vi "Measure EQE.vi"(6 "Skip cell?":bool, 8 "Scan settings":T1={"J-V scan"=TRUE, "J-t scan"=FALSE, "Min voltage (V)"=0.0, "Max voltage (V)"=1.4, "Step (V)"=0.01, "Measurement delay (ms)"=10.0, "1st scan FB-SC"=TRUE, "Inverted structure"=FALSE, "Stabilisation time (s)"=0.0, "Stabilisation mode"=0, "Stabilisation value (V or A) "=0.0, "Step time (s)"=1.0, "Integration time"=0, "Repeat light scans"=FALSE, "Stabilisation in the dark?"=FALSE, "J-t Min (V)"=0.0, "J-t Max (V)"=1.4, "J-t Step (V)"=0.01, "Max. power stabilisation"=FALSE, "J-t 1st scan FB-SC"=TRUE, "J-t Inverted structure"=FALSE, "Max power tracking"=FALSE, "Vmp (V)"=0.7, "Total stabilisation time (s)"=100.0, "J-t best pixel only"=0, "Max power best pixel only"=0, "Vmp from J-V scan"=FALSE, "Intensity dependence"=FALSE, "P dep best pixel only"=0, "External quantum efficiency"=FALSE, "EQE best pixel only"=0, "WL min (nm)"=300.0, "WL max (nm)"=900.0, "WL step (nm)"=5.0, "Wait (ms)"=100.0, "No. of repeat scans"=2.0, "Only repeat for best pixel"=0, "Chopper Freq.  (Hz)"=90.0, "Time Constant (s)"=2.0, "Stabilisation time step (s)"=1.0, "Illumination conditions"=2, "Scan rate min (V/s)"=0.1, "Scan rate max (V/s)"=1.0, "No. of scan rate steps"=1.0, "Scan rate voltage step priority"=FALSE, "Scan rate measurement delay priority"=FALSE, "J-t Illumination conditions"=0, "White bias  (no. of suns)"=200.0, "Max P stab. Specific voltage"=FALSE} {"J-t Illumination conditions" items=["Light only", "Dark only", "Light then dark", "Dark then light"]; "No. of scan rate steps" min=1.0 step=1.0; "Illumination conditions" items=["Light only", "Dark only", "Light then dark", "Dark then light", "Light then dark then light", "Dark then light then dark"]; "Time Constant (s)" items=["0.003", "0.01", "0.03", "0.1", "0.3", "1", "3", "10", "30", "100"]; "Only repeat for best pixel" items=["only for best pixel", "for best 2 pixels", "for best 3 pixels", "for best 4 pixels", "for best 5 pixels", "for best 6 pixels", "for best 7 pixels", "for all pixels"]; "No. of repeat scans" min=1.0 step=1.0; "EQE best pixel only" items=["only the best pixel", "the best 2 pixel", "the best 3 pixel", "the best 4 pixel", "the best 5 pixel", "the best 6 pixel", "the best 7 pixel", "all pixels"]; "P dep best pixel only" items=["only the best pixel", "the best 2 pixels", "the best 3 pixels", "the best 4 pixels", "the best 5 pixels", "the best 6 pixels", "the best 7 pixels", "all pixels"]; "Max power best pixel only" items=["only the best pixel", "the best 2 pixels", "the best 3 pixels", "the best 4 pixels", "the best 5 pixels", "the best 6 pixels", "the best 7 pixels", "all pixels"]; "J-t best pixel only" items=["only the best pixel", "the best 2 pixels", "the best 3 pixels", "the best 4 pixels", "the best 5 pixels", "the best 6 pixels", "the best 7 pixels", "all pixels"]; "Integration time" items=["Fast", "Normal", "High Accuracy"]; "Stabilisation mode" items=["V", "I"]; "Measurement delay (ms)" min=10.0}, 9 "Save data file path":string) -> (0 "Max WL (nm)":string, 1 "Min WL (nm)":string, 3 "EQE data file path":path)   [LabVIEW 2011]
uses:
  TypeDefs/Scan settings.ctl
  TypeDefs/Settings Boolean.ctl
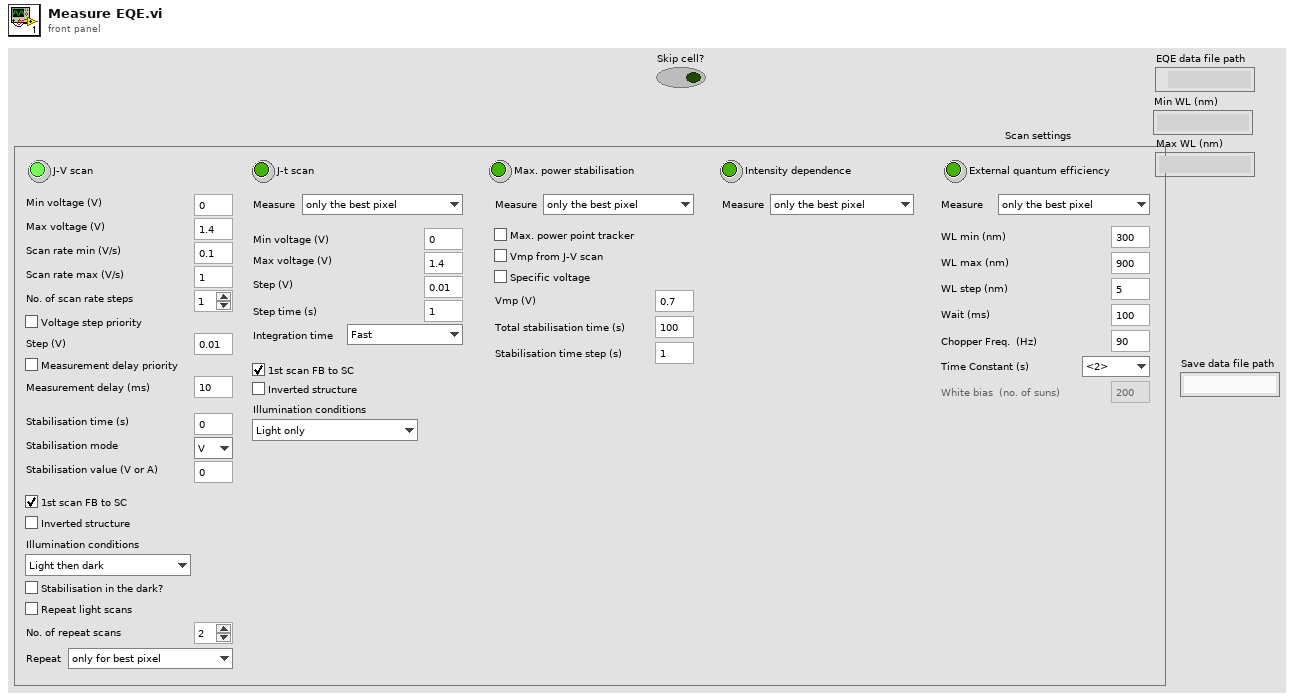
[diagram p1: front panel]
types:
  T1 = typedef "Scan settings.ctl" = cluster{"J-V scan":T2, "J-t scan":bool, "Min voltage (V)":dbl, "Max voltage (V)":dbl, "Step (V)":dbl, "Measurement delay (ms)":dbl, "1st scan FB-SC":bool, "Inverted structure":bool, "Stabilisation time (s)":dbl, "Stabilisation mode":u16, "Stabilisation value (V or A) ":dbl, "Step time (s)":dbl, "Integration time":u16, "Repeat light scans":bool, "Stabilisation in the dark?":bool, "J-t Min (V)":dbl, "J-t Max (V)":dbl, "J-t Step (V)":dbl, "Max. power stabilisation":bool, "J-t 1st scan FB-SC":bool, "J-t Inverted structure":bool, "Max power tracking":bool, "Vmp (V)":dbl, "Total stabilisation time (s)":dbl, "J-t best pixel only":u16, "Max power best pixel only":u16, "Vmp from J-V scan":bool, "Intensity dependence":bool, "P dep best pixel only":u16, "External quantum efficiency":bool, "EQE best pixel only":u16, "WL min (nm)":dbl, "WL max (nm)":dbl, "WL step (nm)":dbl, "Wait (ms)":dbl, "No. of repeat scans":dbl, "Only repeat for best pixel":u16, "Chopper Freq.  (Hz)":dbl, "Time Constant (s)":dbl, "Stabilisation time step (s)":dbl, "Illumination conditions":u16, "Scan rate min (V/s)":dbl, "Scan rate max (V/s)":dbl, "No. of scan rate steps":dbl, "Scan rate voltage step priority":bool, "Scan rate measurement delay priority":bool, "J-t Illumination conditions":u16, "White bias  (no. of suns)":dbl, "Max P stab. Specific voltage":bool}
  T2 = typedef "Settings Boolean.ctl" = bool
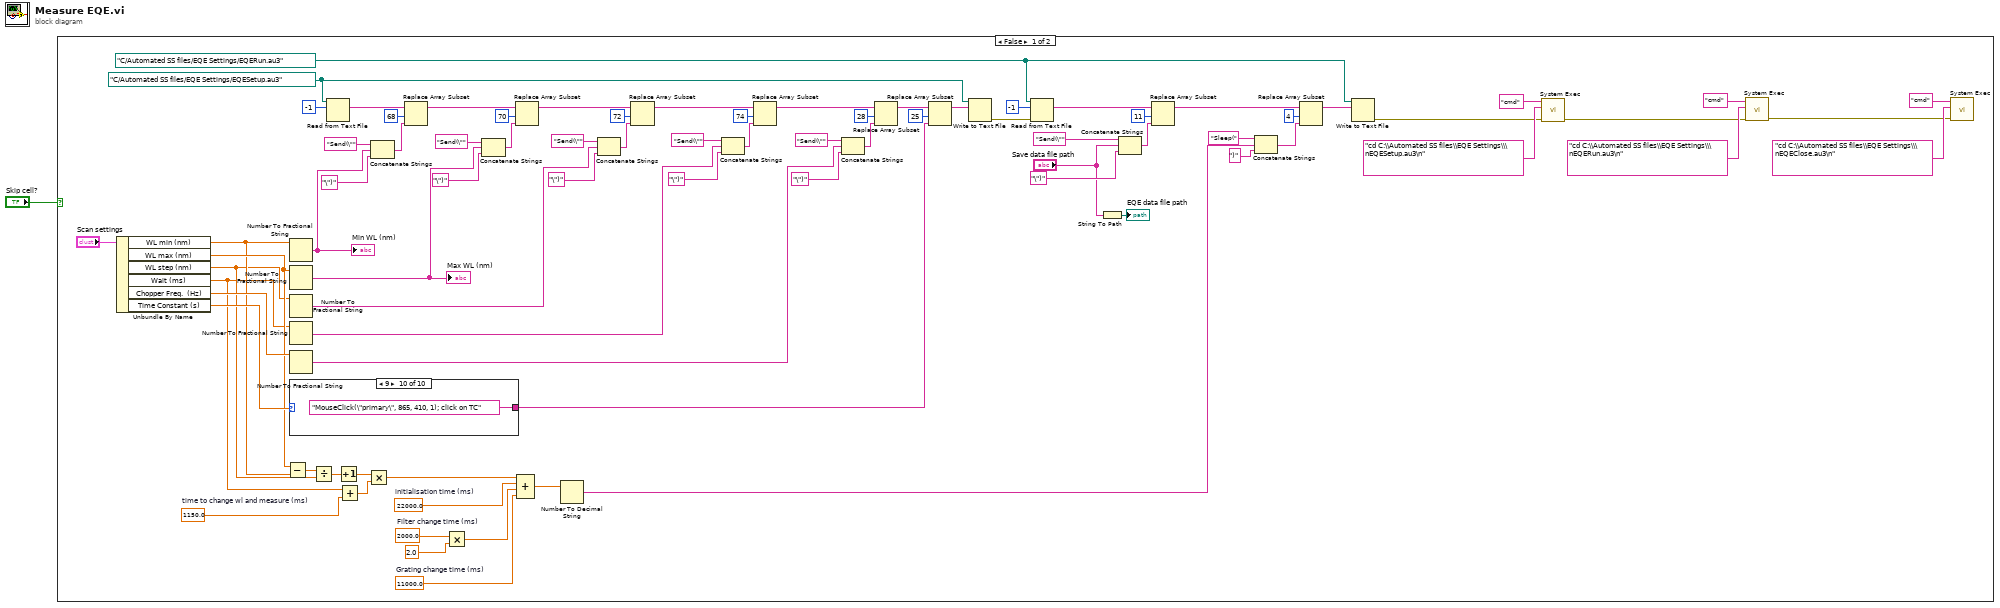
[diagram p0: block diagram]
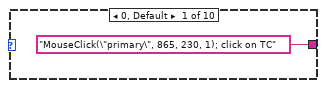
[diagram p2: hidden frame]
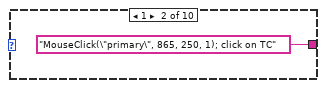
[diagram p3: hidden frame]
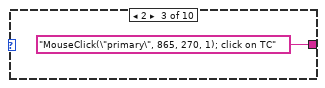
[diagram p4: hidden frame]
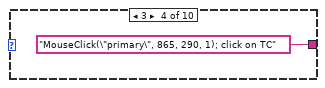
[diagram p5: hidden frame]
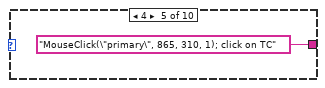
[diagram p6: hidden frame]
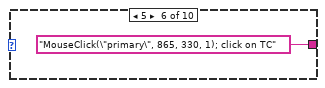
[diagram p7: hidden frame]
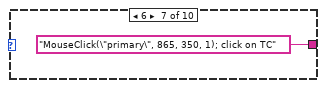
[diagram p8: hidden frame]
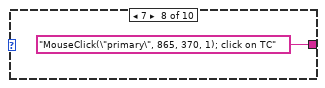
[diagram p9: hidden frame]
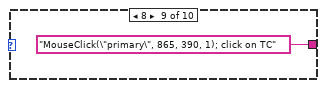
[diagram p10: hidden frame]
diagram:
  n1 = case shown="False" "Skip cell?" {
    frame False {
      w11 = 11000.0  # Grating change time (ms)
      w14 = 2000.0  # Filter change time (ms)
      w15 = 22000.0  # initialisation time (ms)
      w19 = 1150.0  # time to change wl and measure (ms)
      w3 = path "C:/Automated SS files/EQE Settings/EQERun.au3" ("file (use dialog)")
      w54 = path "C:/Automated SS files/EQE Settings/EQESetup.au3" ("file (use dialog)")
      n2 = Unbundle By Name("Scan settings") -> ("WL min (nm)"=w24:dbl, "WL max (nm)"=w25:dbl, "WL step (nm)"=w22:dbl, "Wait (ms)"=w18:dbl, "Chopper Freq.  (Hz)"=w36:dbl, "Time Constant (s)"=w34:dbl)
      n3 = Subtract(x=w25, y=w24) -> (x-y=w23:dbl)
      n4 = Number To Fractional String(number=w24) -> (F-format string=w47:string)  [unwired: 3 in]
      "Min WL (nm)" <- w47
      n5 = Number To Fractional String(number=w25) -> (F-format string=w46:string)  [unwired: 3 in]
      "Max WL (nm)" <- w46
      n6 = Number To Fractional String(number=w22) -> (F-format string=w45:string)  [unwired: 3 in]
      n7 = Number To Fractional String(number=w18) -> (F-format string=w44:string)  [unwired: 3 in]
      n8 = Number To Fractional String(number=w36) -> (F-format string=w35:string)  [unwired: 3 in]
      n9 = case shown="9" w34 {
        tunnel: ["MouseClick(\"primary\", 865, 230, 1); click on TC" ("string") "MouseClick(\"primary\", 865, 250, 1); click on TC" ("string") "MouseClick(\"primary\", 865, 270, 1); click on TC" ("string") "MouseClick(\"primary\", 865, 290, 1); click on TC" ("string") "MouseClick(\"primary\", 865, 310, 1); click on TC" ("string") "MouseClick(\"primary\", 865, 330, 1); click on TC" ("string") "MouseClick(\"primary\", 865, 350, 1); click on TC" ("string") "MouseClick(\"primary\", 865, 370, 1); click on TC" ("string") "MouseClick(\"primary\", 865, 390, 1); click on TC" ("string") "MouseClick(\"primary\", 865, 410, 1); click on TC" ("string")] -> w30
        frame 0, Default {
        }
        frame 1 {
        }
        frame 2 {
        }
        frame 3 {
        }
        frame 4 {
        }
        frame 5 {
        }
        frame 6 {
        }
        frame 7 {
        }
        frame 8 {
        }
        frame 9 {
        }
      }
      n10 = Divide(x=w23, y=w22) -> (x/y=w21:dbl)
      n11 = Read from Text File(file (use dialog)=w54, count=-1) -> (text=w75:string[])  [unwired: 2 in, 3 out]
      n12 = Increment(x=w21) -> (x+1=w20:dbl)
      n13 = Add(x=w18, y=w19) -> (x+y=w17:dbl)
      n14 = Multiply(x=w20, y=w17) -> (x*y=w16:dbl)
      n15 = Concatenate Strings("Send(\"" ("string"), w47, "\")" ("string")) -> (w66:string)
      n16 = Replace Array Subset(array=w75, new element=w66, index=68) -> (w72:string[])
      n17 = Multiply(x=w14, y=2.0) -> (x*y=w12:dbl)
      n18 = Concatenate Strings("Send(\"" ("string"), w46, "\")" ("string")) -> (w61:string)
      n19 = Replace Array Subset(array=w72, new element=w61, index=70) -> (w70:string[])
      n20 = Compound Arithmetic op=ADD(w16, w15, w12, w11) -> (w10:dbl)
      n21 = Number To Decimal String(number=w10) -> (decimal integer string=w8:string)  [unwired: 1 in]
      n22 = Concatenate Strings("Send(\"" ("string"), w45, "\")" ("string")) -> (w58:string)
      n23 = Replace Array Subset(array=w70, new element=w58, index=72) -> (w68:string[])
      n24 = Concatenate Strings("Send(\"" ("string"), w44, "\")" ("string")) -> (w55:string)
      n25 = Replace Array Subset(array=w68, new element=w55, index=74) -> (w37:string[])
      n26 = Concatenate Strings("Send(\"" ("string"), w35, "\")" ("string")) -> (w38:string)
      n27 = Replace Array Subset(array=w37, new element=w38, index=28) -> (w32:string[])
      n28 = Replace Array Subset(array=w32, new element=w30, index=25) -> (w31:string[])
      n29 = Write to Text File(file (use dialog)=w54, text=w31) -> (error out=w4:errorcluster)  [unwired: 2 in, 2 out]
      n30 = Read from Text File(file (use dialog)=w3, count=-1, error in=w4) -> (text=w28:string[])  [unwired: 1 in, 3 out]
      n31 = String To Path(string="Save data file path") -> (path=→"EQE data file path":path)
      n32 = Concatenate Strings("Send(\"" ("string"), "Save data file path", "\")" ("string")) -> (w49:string)
      n33 = Replace Array Subset(array=w28, new element=w49, index=11) -> (w26:string[])
      n34 = Concatenate Strings("Sleep(" ("string"), w8, ")" ("string")) -> (w6:string)
      n35 = Replace Array Subset(array=w26, new element=w6, index=4) -> (w5:string[])
      n36 = Write to Text File(file (use dialog)=w3, text=w5) -> (error out=w2:errorcluster)  [unwired: 2 in, 2 out]
      n37 = call <vilib>:"System Exec.vi"("error in (no error)"=w2, "standard input"="cd C:\\Automated SS files\\EQE Settings\\\nEQESetup.au3\n", "command line"="cmd") -> ("error out"=w53:errorcluster)  [unwired: 5 in, 3 out]
      n38 = call <vilib>:"System Exec.vi"("error in (no error)"=w53, "standard input"="cd C:\\Automated SS files\\EQE Settings\\\nEQERun.au3\n", "command line"="cmd") -> ("error out"=w76:errorcluster)  [unwired: 5 in, 3 out]
      n39 = call <vilib>:"System Exec.vi"("error in (no error)"=w76, "standard input"="cd C:\\Automated SS files\\EQE Settings\\\nEQEClose.au3\n", "command line"="cmd") -> ()  [unwired: 5 in, 4 out]
    }
    frame True {
    }
  }
